vi "1.标记数据集.vi"() -> ()   [LabVIEW 2013]
uses:
  <vilib>/vision/Image Controls.llb/IMAQ Image.ctl
  <vilib>/vision/Avi.llb/IMAQ AVI2 Refnum.ctl
panel:
  out "标记数据集状态":T1
  in  "关闭":bool
  out "有按键按下":bool
  out "原图":T2(plugin-control)
  in  "帧率":dbl=1.0 min=1.0 max=1000.0
  out "状态":T1
  in  "视频文件路径":path
  in  "浏览":bool
  in  "保存结束帧":bool
  out "第N帧":u32
  in  "微调":i64(slide) scale=-20.0..20.0
  in  "保存起始帧":bool
  in  "停止":bool
  in  "播放":bool
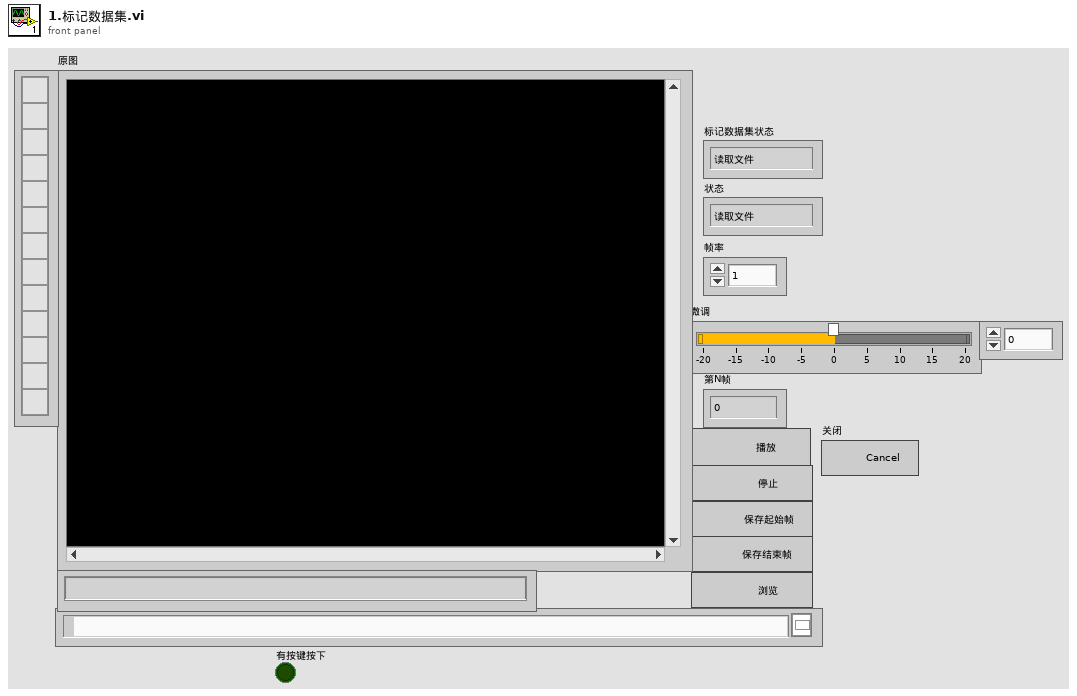
[diagram p1: front panel]
types:
  T1 = typedef "标记数据集状态.ctl" = enum16{"读取文件", "自动播放", "手动微调", "记录起始帧", "记录结束帧", "空闲"}
  T2 = typedef "IMAQ Image.ctl" = refnum<image>
  T3 = typedef "IMAQ AVI2 Refnum.ctl" = refnum<k20>
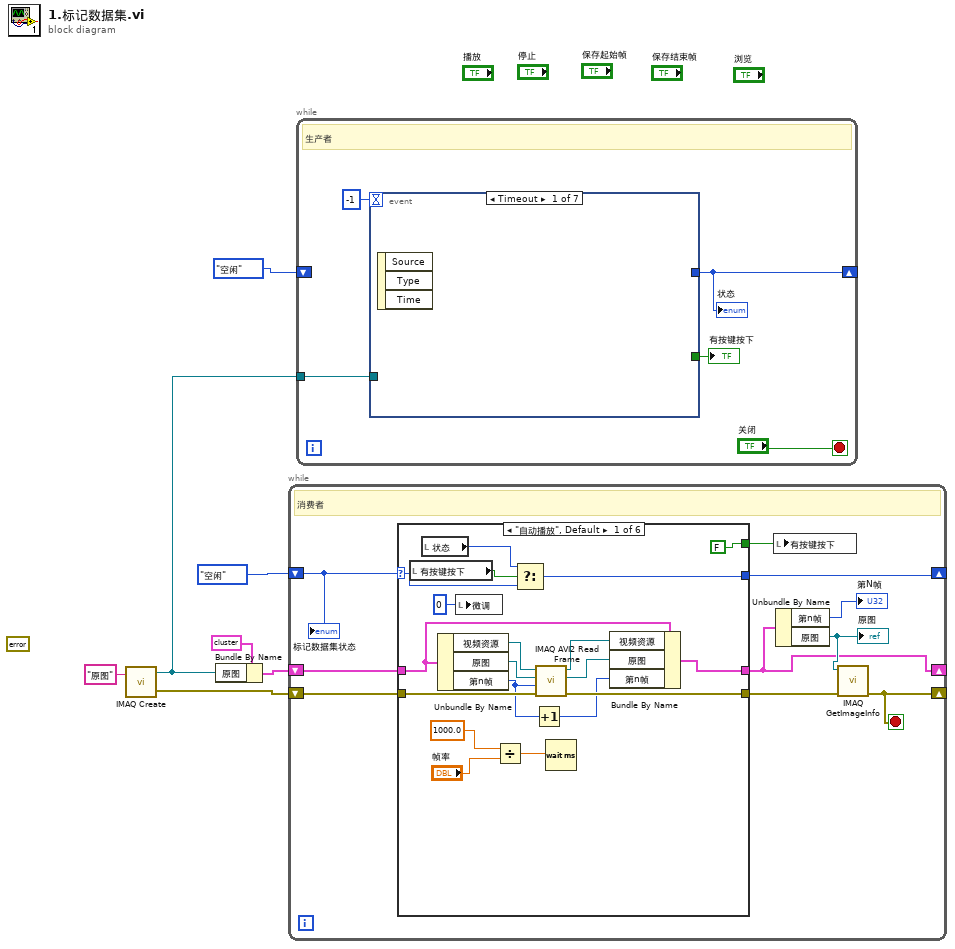
[diagram p0: block diagram]
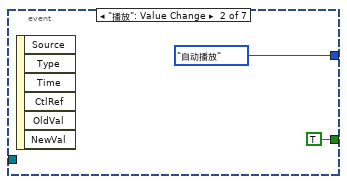
[diagram p2: hidden frame]
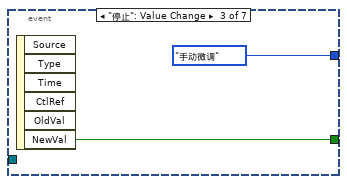
[diagram p3: hidden frame]
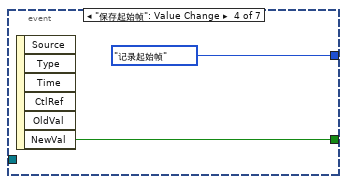
[diagram p4: hidden frame]
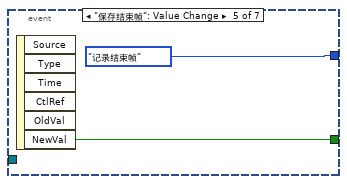
[diagram p5: hidden frame]
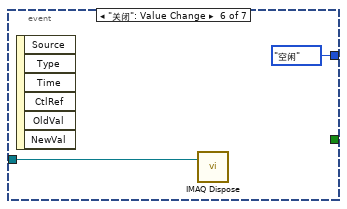
[diagram p6: hidden frame]
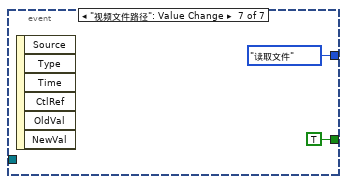
[diagram p7: hidden frame]
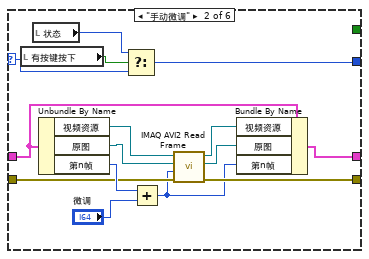
[diagram p8: hidden frame]
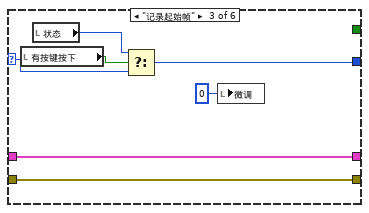
[diagram p9: hidden frame]
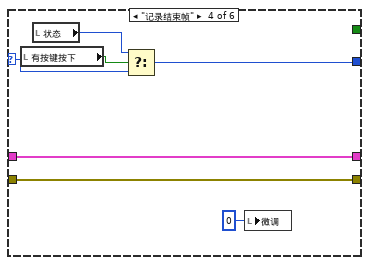
[diagram p10: hidden frame]
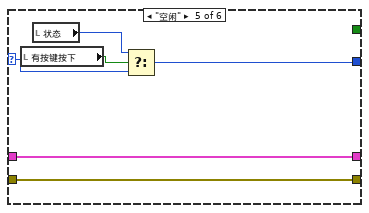
[diagram p11: hidden frame]
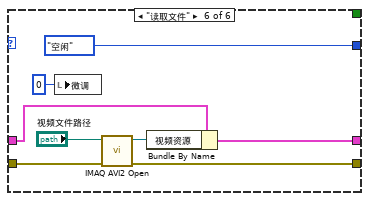
[diagram p12: hidden frame]
diagram:
  (unwired) errorcluster {"status"=FALSE, "code"=0, "source"=""} ("错误簇")
  n1 = call "IMAQ Create"("Image Name"="原图") -> ("New Image"=w2:T2, "error out"=w3:errorcluster)  [unwired: 4 in]
  n2 = Bundle By Name(cluster=cluster{"原图":T2, "视频资源":T3, "第n帧":u32} {"原图"=refnum, "视频资源"=refnum, "第n帧"=0}, "原图"=w2) -> (w4:cluster{"原图":T2, "视频资源":T3, "第n帧":u32})
  n3 = while {
    shift-right: [w16] -> _
    shift-left: 标记数据集状态."空闲" ("标记数据集状态") -> [w17]
    shift-right: [w10] -> _
    shift-left: w4 -> [w15]
    shift-right: [w9] -> _
    shift-left: w3 -> [w14]
    stop <- w9 stop-if-true
    # "消费者"
    n4 = case shown="\"自动播放\", Default" w17 {
      selector: w17 -> [w22 w48 w54 w62 w66 _]
      tunnel: [w23 w49 w55 w61 w67 标记数据集状态."空闲" ("标记数据集状态")] -> w16
      tunnel: w15 -> [w33 w42 w53 w60 w71 w75]
      tunnel: w14 -> [w36 w43 w52 w59 w70 w77]
      tunnel: [w29 w40 w52 w59 w70 w76] -> w12
      tunnel: [w32 w41 w53 w60 w71 w73] -> w10
      tunnel: [FALSE ("有按键按下") _ _ _ _ _] -> w8
      frame "自动播放", Default {
        n5 = local read "有按键按下"() -> (w21:bool)
        n6 = local read "状态"() -> (w20:T1)
        n7 = Unbundle By Name(w33) -> ("视频资源"=w35:T3, "原图"=w34:T2, "第n帧"=w28:u32)
        n8 = local write "微调"(0 ("微调")) -> ()
        n9 = Divide(x=1000.0, y="帧率") -> (x/y=w26:dbl)
        n10 = Select(t=w20, s=w21, f=w22) -> (s? t:f=w23:T1)
        n11 = Increment(x=w28) -> (x+1=w27:u32)
        n12 = call "IMAQ AVI2 Read Frame"("error in (no error)"=w36, "Frame Number"=w28, "Image"=w34, "AVI Refnum"=w35) -> ("error out"=w29:errorcluster, "Image Out"=w30:T2, "AVI Refnum (duplicate)"=w31:T3)  [unwired: 5 in]
        n13 = Wait (ms)(milliseconds to wait=w26) -> ()  [unwired: 1 out]
        n14 = Bundle By Name(cluster=w33, "视频资源"=w31, "原图"=w30, "第n帧"=w27) -> (w32:cluster{"原图":T2, "视频资源":T3, "第n帧":u32})
      }
      frame "手动微调" {
        n15 = local read "有按键按下"() -> (w51:bool)
        n16 = local read "状态"() -> (w50:T1)
        n17 = Unbundle By Name(w42) -> ("视频资源"=w47:T3, "原图"=w46:T2, "第n帧"=w45:u32)
        n18 = Select(t=w50, s=w51, f=w48) -> (s? t:f=w49:T1)
        n19 = Add(x=w45, y="微调") -> (x+y=w37:i64)
        n20 = call "IMAQ AVI2 Read Frame"("error in (no error)"=w43, "Frame Number"=w37, "Image"=w46, "AVI Refnum"=w47) -> ("error out"=w40:errorcluster, "Image Out"=w38:T2, "AVI Refnum (duplicate)"=w39:T3)  [unwired: 5 in]
        n21 = Bundle By Name(cluster=w42, "视频资源"=w39, "原图"=w38, "第n帧"=w37) -> (w41:cluster{"原图":T2, "视频资源":T3, "第n帧":u32})
      }
      frame "记录起始帧" {
        n22 = local read "有按键按下"() -> (w57:bool)
        n23 = local read "状态"() -> (w56:T1)
        n24 = Select(t=w56, s=w57, f=w54) -> (s? t:f=w55:T1)
        n25 = local write "微调"(0 ("微调")) -> ()
      }
      frame "记录结束帧" {
        n26 = local read "有按键按下"() -> (w64:bool)
        n27 = local read "状态"() -> (w63:T1)
        n28 = Select(t=w63, s=w64, f=w62) -> (s? t:f=w61:T1)
        n29 = local write "微调"(0 ("微调")) -> ()
      }
      frame "空闲" {
        n30 = local read "有按键按下"() -> (w69:bool)
        n31 = local read "状态"() -> (w68:T1)
        n32 = Select(t=w68, s=w69, f=w66) -> (s? t:f=w67:T1)
      }
      frame "读取文件" {
        n33 = local write "微调"(0 ("微调")) -> ()
        n34 = call "IMAQ AVI2 Open"("error in (no error)"=w77, "AVI File Path"="视频文件路径") -> ("error out"=w76:errorcluster, "AVI Refnum"=w74:T3)  [unwired: 8 in]
        n35 = Bundle By Name(cluster=w75, "视频资源"=w74) -> (w73:cluster{"原图":T2, "视频资源":T3, "第n帧":u32})
      }
    }
    n36 = local write "有按键按下"(w8) -> ()
    n37 = Unbundle By Name(w10) -> ("第n帧"=→"第N帧":u32, "原图"=w11:T2)
    "原图" <- w11
    n38 = call "IMAQ GetImageInfo"("error in (no error)"=w12, "Image"=w11) -> ("error out"=w9:errorcluster)  [unwired: 2 in, 7 out]
    "标记数据集状态" <- w17
  }
  n39 = while {
    tunnel: w2 -> [w82]
    shift-right: [w80] -> _
    shift-left: 标记数据集状态."空闲" ("标记数据集状态") -> [_]
    stop <- "关闭" stop-if-true
    # "生产者"
    n40 = event shown="[0] Timeout" {
      selector: _ -> [_ _ _ _ _ _ _]
      dyn-events: _ -> [_ _ _ _ _ _ _]
      timeout: -1 -> [_ _ _ _ _ _ _]
      tunnel: [_ 标记数据集状态."自动播放" ("标记数据集状态") 标记数据集状态."手动微调" ("标记数据集状态") 标记数据集状态."记录起始帧" ("标记数据集状态") 标记数据集状态."记录结束帧" ("标记数据集状态") 标记数据集状态."空闲" ("标记数据集状态") 标记数据集状态."读取文件" ("标记数据集状态")] -> w80
      tunnel: [_ TRUE ("NewVal") w87 w89 w91 _ TRUE ("NewVal")] -> w84
      tunnel: w82 -> [_ _ _ _ _ w94 _]
      event Timeout {
        n41 = event-data() -> ()  [unwired: 1 in, 3 out]
      }
      event "播放": Value Change {
        n42 = event-data() -> ()  [unwired: 1 in, 6 out]
      }
      event "停止": Value Change {
        n43 = event-data() -> ("NewVal"=w87:bool)  [unwired: 1 in, 5 out]
      }
      event "保存起始帧": Value Change {
        n44 = event-data() -> ("NewVal"=w89:bool)  [unwired: 1 in, 5 out]
      }
      event "保存结束帧": Value Change {
        n45 = event-data() -> ("NewVal"=w91:bool)  [unwired: 1 in, 5 out]
      }
      event "关闭": Value Change {
        n46 = event-data() -> ()  [unwired: 1 in, 6 out]
        n47 = call "IMAQ Dispose"("Image"=w94) -> ()  [unwired: 5 in, 1 out]
      }
      event "视频文件路径": Value Change {
        n48 = event-data() -> ()  [unwired: 1 in, 6 out]
      }
    }
    "状态" <- w80
    "有按键按下" <- w84
  }
